vi "applyAOSCorrectionByBendingModes.vi"(8 "error in (no error)":errorcluster, 10 "Parameters":T1, 11 "Context in":refnum<class "Context.lvclass">) -> (0 "error out":errorcluster, 3 "Context out":refnum<class "Context.lvclass">)   [LabVIEW 2016, in "Context.lvclass"]
uses:
  Context.lvclass
  DataTypes/Topics/CommandApplyAOSCorrectionByBendingModes.ctl
  DataTypes/Topics/Parts/CommandId.ctl
  Context.lvclass/Context.ctl
  States/State/State.lvclass
  Model/Model.lvclass
  DataTypes/Topics/M1M3SupportTopics.lvlib
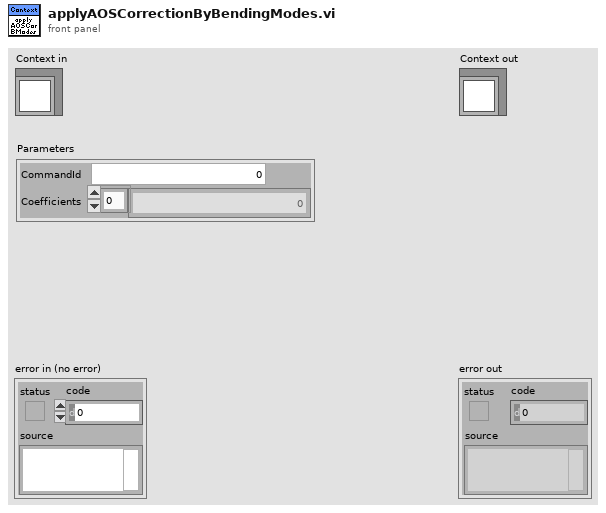
[diagram p1: front panel]
types:
  T1 = typedef "M1M3SupportTopics.lvlib/CommandApplyAOSCorrectionByBendingModes.ctl" = cluster{"CommandId":T2, "Coefficients":dbl[]}
  T2 = typedef "M1M3SupportTopics.lvlib/CommandId.ctl" = i32
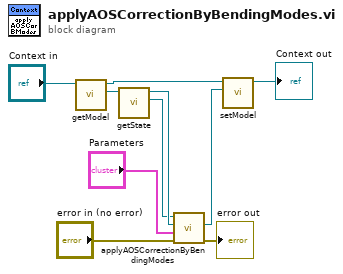
[diagram p0: block diagram]
diagram:
  n1 = call "getModel.vi"("Context in"="Context in") -> ("Model"=w9:refnum<class "Model.lvclass">, "Context out"=w8:refnum<class "Context.lvclass">)  [unwired: 9 in]
  n2 = call "getState.vi"("Model in"=w9) -> ("State out"=w4:refnum<class "State.lvclass">, "Model out"=w5:refnum<class "Model.lvclass">)  [unwired: 8 in, 1 out]
  n3 = call-dynamic "applyAOSCorrectionByBendingModes.vi"("error in (no error)"="error in (no error)", "Parameters"="Parameters", "Model in"=w5, "State in"=w4) -> ("error out"=→"error out":errorcluster, "Model out"=w3:refnum<class "Model.lvclass">)  [unwired: 5 in, 1 out]
  n4 = call "setModel.vi"("Model"=w3, "Context in"=w8) -> ("Context out"=→"Context out":refnum<class "Context.lvclass">)  [unwired: 9 in]
